vi "LoadSet.vi"(9 "File Name In":string, 10 "output array":string[][](array[string])) -> (0 "File Name out":string, 2 "Accepted":bool)   [LabVIEW 2014, in "Panels.lvlib"]
uses:
  Panels.lvlib
  <vilib>/printing/EasyPrintingControls.llb/layout_options.ctl
  <vilib>/printing/EasyPrintingControls.llb/orientation.ctl
  <vilib>/printing/EasyPrintingControls.llb/panel_scaling_for_page.ctl
  <vilib>/printing/EasyPrintingControls.llb/margins.ctl
  <vilib>/printing/EasyPrintingControls.llb/margin_values.ctl
  <vilib>/printing/EasyPrintingControls.llb/measurement_system.ctl
  <vilib>/printing/EasyPrintingControls.llb/printer_options.ctl
  <vilib>/printing/EasyPrintingControls.llb/printing_method.ctl
  <vilib>/printing/EasyPrintingControls.llb/color_or_monochrome.ctl
  <vilib>/printing/EasyPrintingControls.llb/page_header_options.ctl
  <vilib>/printing/EasyPrintingControls.llb/page_headers.ctl
  <vilib>/printing/EasyPrintingControls.llb/page_header_content_options.ctl
  CS_Core/CSSystem/CoreDefs/CoreDefs.call_type.ctl
  CS_Core/BaseProcess/BaseProcess.descriptor string definition.ctl
  CS_Core/CSSystem/CoreDefs/CoreDefs.rawDataType.ctl
  <vilib>/printing/EasyPrintingControls.llb/contents.ctl
  CS_Core/CSSystem/CoreLib/CoreLib.short 2 byte array.vi
  CS_Core/CSSystem/CoreLib/CoreLib.double 2 byte array.vi
  CS_Core/CSSystem/CoreLib/CoreLib.string 2 byte array.vi
  <vilib>/printing/EasyPrinting.llb/Easy Print VI Panel or Documentation (path).vi
  <vilib>/Utility/NIReport.llb/NI_ReportGenerationCore.lvlib
  CS_Core/CSSystem/CoreLib/CoreLib.lvlib
  CS_Core/BaseProcess/BaseProcess.lvlib
panel:
  in  "call cluster in":T1={"Object"="", "Selector"="", "CallType"=enum."synchronous", "Async Object"="", "Async Selector"="", "Data Descriptor"="", "Data"=[], "Error #"=0, "Expire"=0}
  in  "Print":bool
  in  "layout options":T4={"orientation (unchanged)"=0, "panel scaling for page (unchanged)"=0, "margins"={"override VI margins (false)"=FALSE, "margins (1.00)"={"top"=1.0, "left"=1.0, "right"=1.0, "bottom"=1.0}, "measurement system (default)"=0}, "printer options"={"destination printer name (current)"="\\\\Trunk\\WAGNER_PRINT", "printing method (unchanged)"=0, "color or monochrome (unchanged)"=0}, "page header options"={"page headers (unchanged)"=2, "page header content options"={"Include VI Name"=FALSE, "Include VI Path"=FALSE, "Include Last Modification Date"=FALSE, "Include Date Printed"=FALSE, "Include Page Number"=FALSE, "Include VI Icon"=FALSE}}} {"page header options"."page headers (unchanged)" items=["Unchanged", "Include page headers", "Do not include page headers"]; "printer options"."color or monochrome (unchanged)" items=["Unchanged", "Color/grayscale", "Monochrome"]; "printer options"."printing method (unchanged)" items=["Unchanged", "Standard", "PostScript", "Bitmap"]; "panel scaling for page (unchanged)" items=["Unchanged", "No Scaling", "Scale front panel to fit"]; "orientation (unchanged)" items=["Unchanged", "portrait", "landscape"]; "margins"."measurement system (default)" items=["Default", "US", "Metric"]; "margins"."margins (1.00)"."right" format="%.2f"; "margins"."margins (1.00)"."bottom" format="%.2f"; "margins"."margins (1.00)"."top" format="%.2f"; "margins"."margins (1.00)"."left" format="%.2f"}
  in  "No action":bool
  in  "Apply loaded values":bool
  out "Table for loading values":string[][](array[string]) caption="080410_iis2bob5_5keV.set"
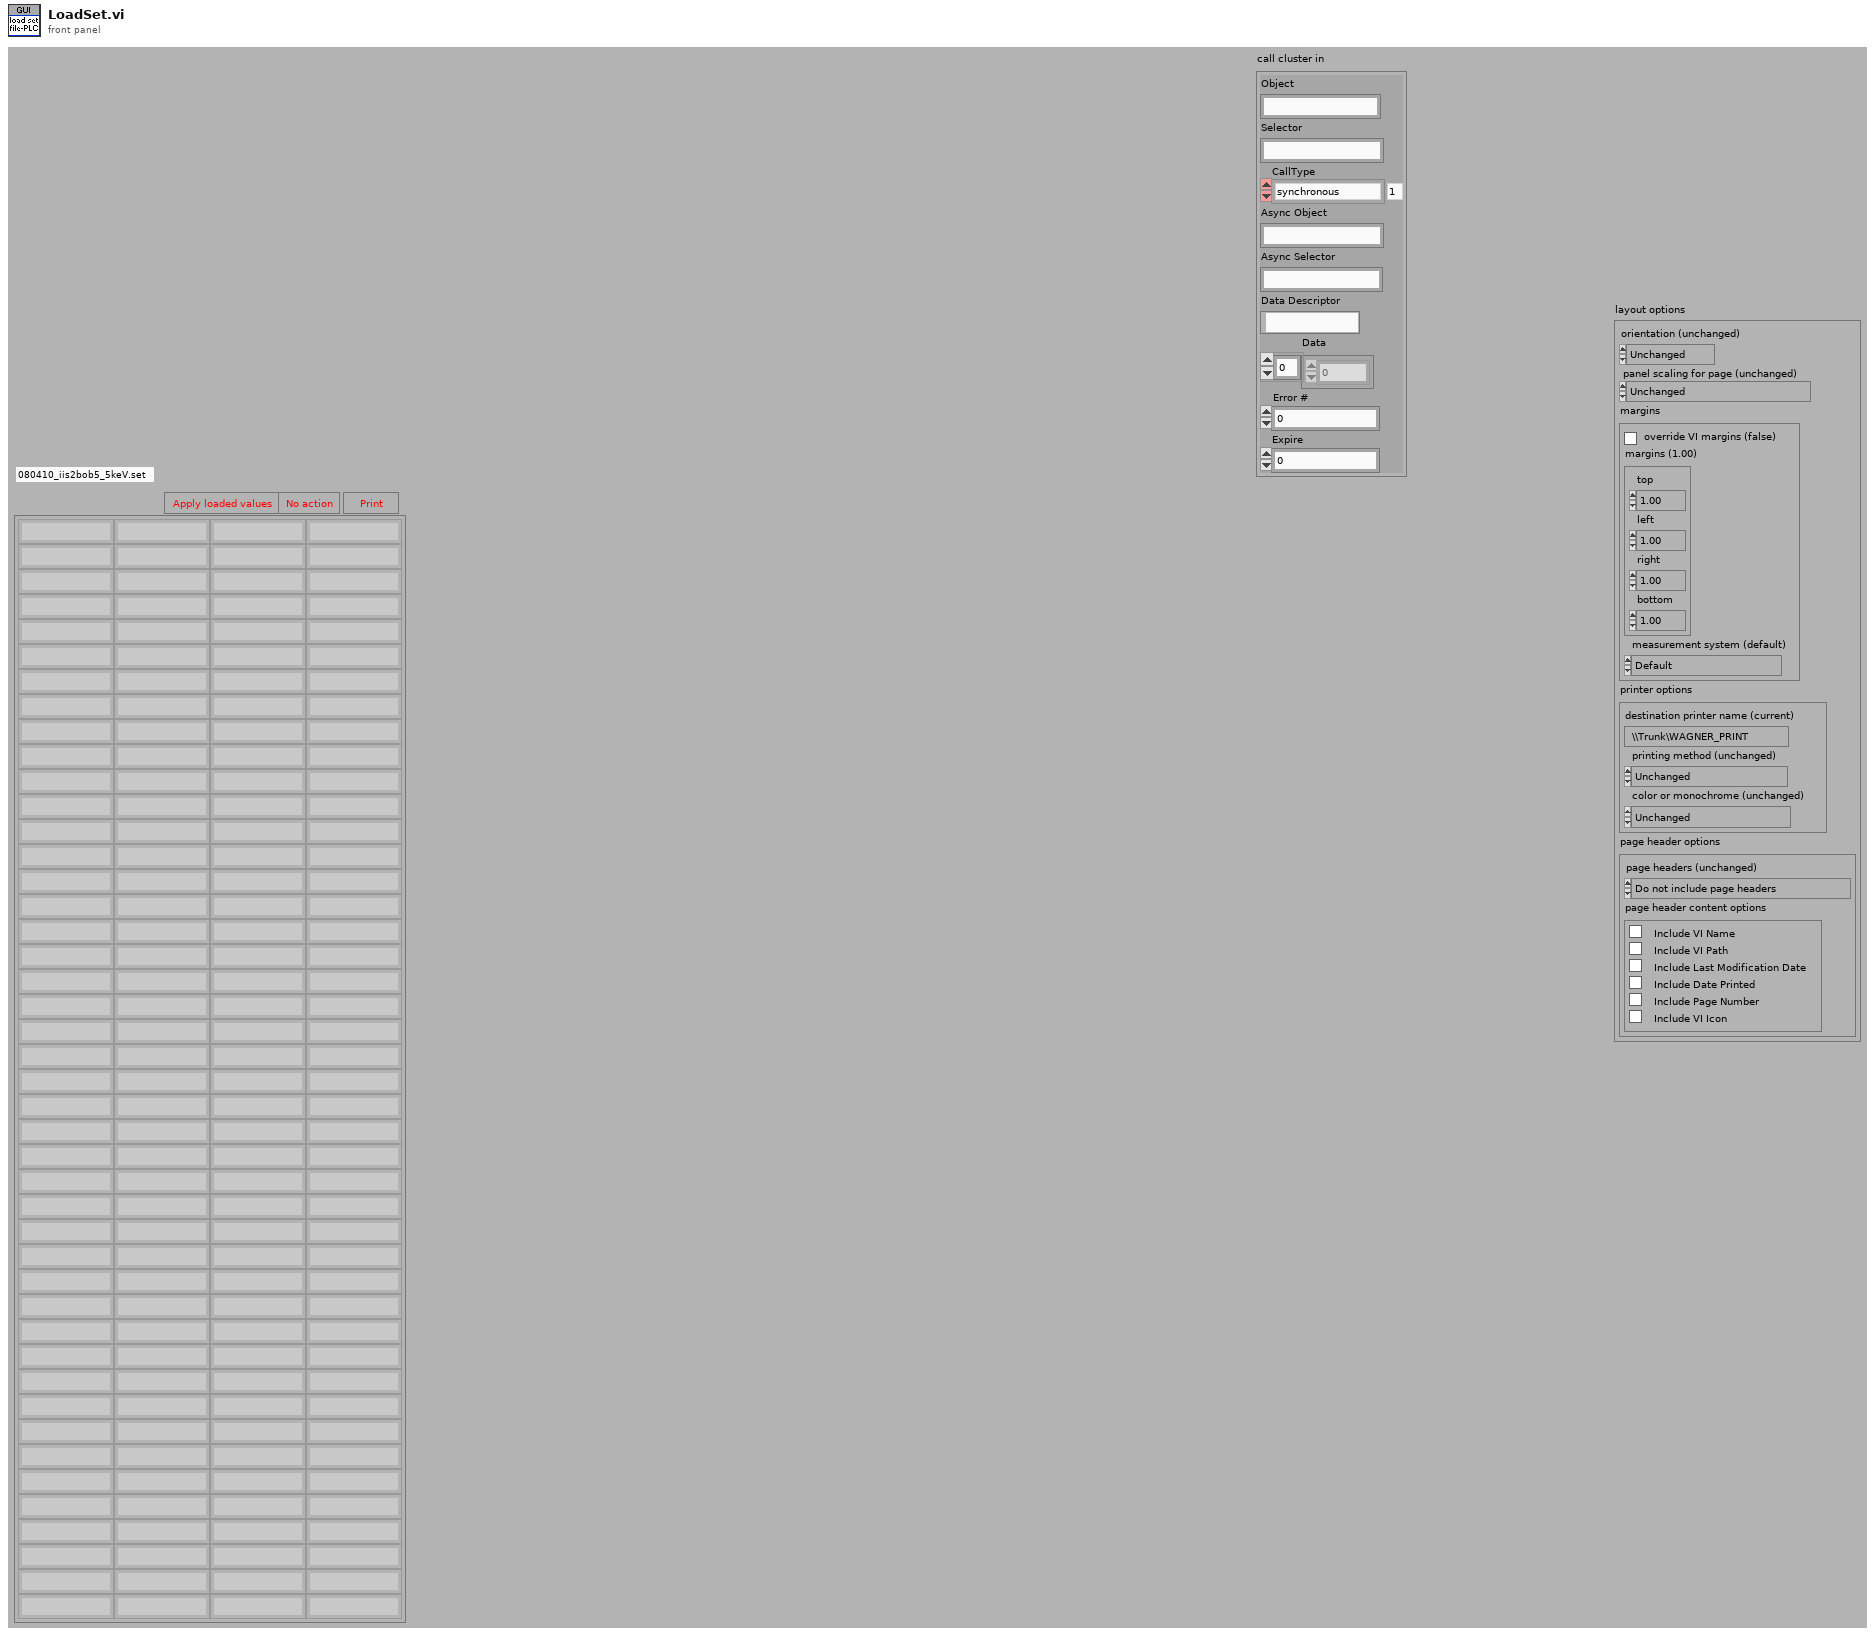
[diagram p1: front panel]
types:
  T1 = typedef "CoreDefs.call_type.ctl" = cluster{"Object":string, "Selector":string, "CallType":enum16{"simple", "synchronous", "asynchronous"}, "Async Object":string, "Async Selector":string, "Data Descriptor":T2, "Data":T3, "Error #":i32, "Expire":u32}
  T2 = typedef "BaseProcess.lvlib/BaseProcess.descriptor string definition.ctl" = string
  T3 = typedef "CoreDefs.rawDataType.ctl" = i8[]
  T4 = typedef "NI_ReportGenerationCore.lvlib/layout_options.ctl" = cluster{"orientation (unchanged)":T5, "panel scaling for page (unchanged)":T6, "margins":T7, "printer options":T10, "page header options":T13}
  T5 = typedef "NI_ReportGenerationCore.lvlib/orientation.ctl" = u16
  T6 = typedef "NI_ReportGenerationCore.lvlib/panel_scaling_for_page.ctl" = u16
  T7 = typedef "NI_ReportGenerationCore.lvlib/margins.ctl" = cluster{"override VI margins (false)":bool, "margins (1.00)":T8, "measurement system (default)":T9}
  T8 = typedef "NI_ReportGenerationCore.lvlib/margin_values.ctl" = cluster{"top":dbl, "left":dbl, "right":dbl, "bottom":dbl}
  T9 = typedef "NI_ReportGenerationCore.lvlib/measurement_system.ctl" = u16
  T10 = typedef "NI_ReportGenerationCore.lvlib/printer_options.ctl" = cluster{"destination printer name (current)":string, "printing method (unchanged)":T11, "color or monochrome (unchanged)":T12}
  T11 = typedef "NI_ReportGenerationCore.lvlib/printing_method.ctl" = u16
  T12 = typedef "NI_ReportGenerationCore.lvlib/color_or_monochrome.ctl" = u16
  T13 = typedef "NI_ReportGenerationCore.lvlib/page_header_options.ctl" = cluster{"page headers (unchanged)":T14, "page header content options":T15}
  T14 = typedef "NI_ReportGenerationCore.lvlib/page_headers.ctl" = u16
  T15 = typedef "NI_ReportGenerationCore.lvlib/page_header_content_options.ctl" = cluster{"Include VI Name":bool, "Include VI Path":bool, "Include Last Modification Date":bool, "Include Date Printed":bool, "Include Page Number":bool, "Include VI Icon":bool}
  T16 = typedef "LVRectTypeDef.ctl" = cluster{"Left":i16, "Top":i16, "Right":i16, "Bottom":i16}
  T17 = typedef "LVBoundsTypeDef.ctl" = cluster{"Width":u32, "Height":u32}
  T18 = typedef "NI_ReportGenerationCore.lvlib/contents.ctl" = u16
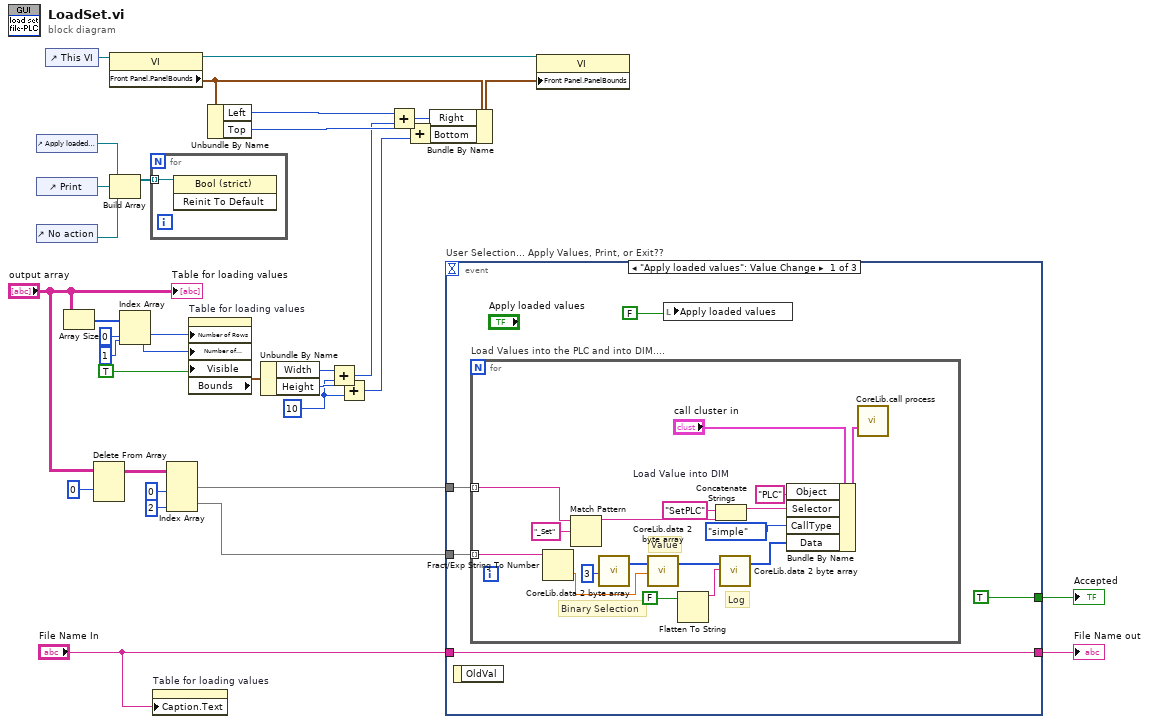
[diagram p0: block diagram]
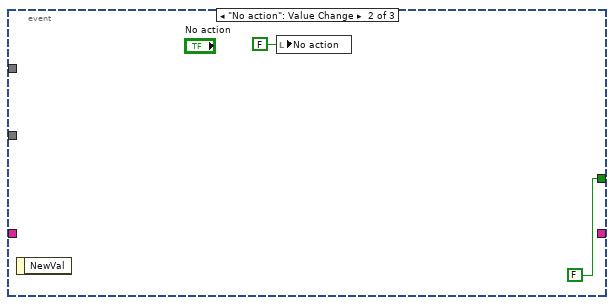
[diagram p2: hidden frame]
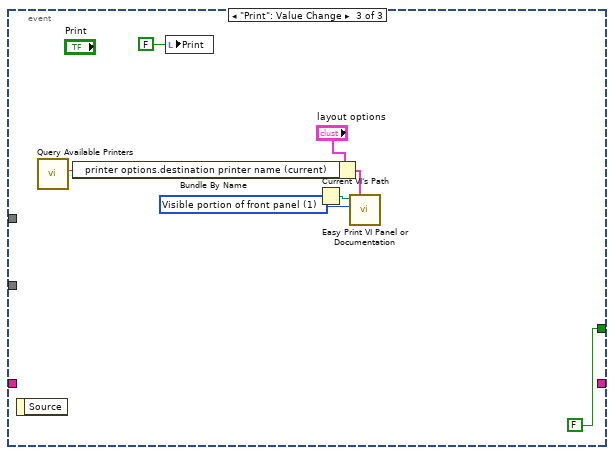
[diagram p3: hidden frame]
diagram:
  w3 = u32 10 ("y")
  n1 = control-ref of="Apply loaded values"() -> (w17:refnum<vi>)
  n2 = control-ref of="Print"() -> (w16:refnum<vi>)
  n3 = control-ref of="No action"() -> (w15:refnum<vi>)
  n4 = control-ref of="This VI"() -> (w14:refnum<vi>)
  n5 = Array Size(array="output array") -> (size(s)=w34:i32[])
  n6 = Delete From Array(array="output array", index (row)=0) -> (array with subset deleted=w25:string[][])  [unwired: 2 in, 1 out]
  n7 = property class="VI"(reference=w14) -> (reference out=w7:refnum<vi>, "Front Panel.PanelBounds"=w10:T16)  [unwired: 1 in, 1 out]
  n8 = Build Array(w17, w16, w15) -> (w18:refnum<vi>[])
  n9 = Index Array(array=w34, index #1=0 ("index"), index #2=1 ("index")) -> (element #1=w33:i32, element #2=w29:i32)
  n10 = for {
    tunnel: w18 -> [w35] mode=indexing
    n11 = invoke class="Bool (strict)" method="Reinit To Default"(reference=w35) -> ()  [unwired: 2 in, 3 out]
  }
  n12 = property on="Table for loading values" class="Arr (strict)"("Caption.Text"="File Name In") -> ()  [unwired: 2 in, 2 out]
  n13 = Index Array(array=w25, index (col) #1=0 ("disabled index (col)"), index (col) #2=2 ("index (col)")) -> (element #1=w23:string[], element #2=w22:string[])  [unwired: 2 in]
  n14 = property on="Table for loading values" class="Arr (strict)"("Number of Rows"=w33, "Number of Columns"=w29, "Visible"=TRUE) -> ("Bounds"=w13:T17)  [unwired: 2 in, 2 out]
  n15 = Unbundle By Name(w10) -> ("Left"=w12:i16, "Top"=w11:i16)
  n16 = Unbundle By Name(w13) -> ("Width"=w4:u32, "Height"=w5:u32)
  n17 = Add(x=w4, y=w3) -> (x+y=w2:u32)
  n18 = Add(x=w5, y=w3) -> (x+y=w1:u32)
  n19 = Add(x=w12, y=w2) -> (x+y=w9:u32)
  n20 = Add(x=w11, y=w1) -> (x+y=w8:u32)
  n21 = Bundle By Name(cluster=w10, "Right"=w9, "Bottom"=w8) -> (w6:T16)
  n22 = event "User Selection... Apply Values, Print, or Exit??" shown="[0] \"Apply loaded values\": Value Change" {
    selector: _ -> [_ _ _]
    dyn-events: _ -> [_ _ _]
    timeout: _ -> [_ _ _]
    tunnel: w23 -> [w39 _ _]
    tunnel: w22 -> [w38 _ _]
    tunnel: "File Name In" -> [w37 _ _]
    tunnel: [w37 _ _] -> w20
    tunnel: [TRUE FALSE FALSE] -> w19
    event "Apply loaded values": Value Change {
      n23 = event-data() -> ()  [unwired: 1 in, 1 out]
      n24 = for "Load Values into the PLC and into DIM...." {
        tunnel: w39 -> [w57] mode=indexing
        tunnel: w38 -> [w56] mode=indexing
        w53 = "PLC"  # Load Value into DIM
        # "Log"
        # "Value"
        # "Binary Selection"
        n25 = Fract/Exp String To Number(string=w56) -> (number=w43:dbl)  [unwired: 3 in, 1 out]
        n26 = Match Pattern(string=w57, regular expression="_Set") -> (before substring=w48:string)  [unwired: 1 in, 3 out]
        n27 = call-poly "CoreLib.data 2 byte array.vi"("i16"=i16 3 ("f64")) -> ("byteArray out"=w42:T3)  [unwired: 18 in]
        n28 = call-poly "CoreLib.data 2 byte array.vi"("byteArray"=w42, "f64"=w43) -> ("byteArray out"=w45:T3)  [unwired: 17 in]
        n29 = Flatten To String(anything=FALSE) -> (data string=w47:string)  [unwired: 3 in, 2 out]
        n30 = Concatenate Strings("SetPLC" ("string"), w48) -> (w51:string)
        n31 = call-poly "CoreLib.data 2 byte array.vi"("byteArray"=w45, "string"=w47) -> ("byteArray out"=w46:T3)  [unwired: 17 in]
        n32 = Bundle By Name(cluster="call cluster in", "Object"=w53, "Selector"=w51, "CallType"=enum16{"simple", "synchronous", "asynchronous"}."simple", "Data"=w46) -> (w54:T1)
        n33 = call "CoreLib.call process.vi"("call cluster in"=w54) -> ()  [unwired: 13 in, 2 out]
      }
      n34 = local write "Apply loaded values"(FALSE ("Apply loaded values")) -> ()
    }
    event "No action": Value Change {
      n35 = event-data() -> ()  [unwired: 1 in, 1 out]
      n36 = local write "No action"(FALSE ("No action")) -> ()
    }
    event "Print": Value Change {
      w64 = T18 1 items=["Complete front panel", "Visible portion of front panel", "Icon, description, panel and diagram", "Documentation: Using the panel", "Documentation: Using as a subVI", "Documentation: Complete", "Documentation: Custom"] ("contents (complete front panel)")
      n37 = event-data() -> ()  [unwired: 1 in, 1 out]
      n38 = call <vilib>:"Query Available Printers.vi"() -> ("default printer"=w62:string)  [unwired: 9 in, 2 out]
      n39 = Bundle By Name(cluster="layout options", "printer options.destination printer name (current)"=w62) -> (w61:T4)
      n40 = local write "Print"(FALSE ("Print")) -> ()
      n41 = Current VI's Path() -> (path=w65:path)
      n42 = call-poly <vilib>:"Easy Print VI Panel or Documentation.vi"("layout options"=w61, "contents (complete front panel)"=w64, "VI path"=w65) -> ()  [unwired: 7 in, 2 out]
    }
  }
  "File Name out" <- w20
  "Accepted" <- w19
  n43 = property class="VI"(reference=w7, "Front Panel.PanelBounds"=w6) -> ()  [unwired: 1 in, 2 out]
  "Table for loading values" <- "output array"
